vi "Bridge Panel.vi"(8 "error in":errorcluster, 11 "bridge in":T3={"type"=enum."TWM client", "TWM"={"pipe name"="", "parameters"=[], "handle"=0, "fixed aper [s]"=0.0, "f-list [Hz]"=[], "discrete f-list"=FALSE, "unc mode"=enum."None", "unc mcc"=0, "unc first"=FALSE}, "last f"=0.0, "bias comp"={"bias type"=enum."dummy", "VISA"="", "Enable"=FALSE, "channel qu"=[], "channel Uinit"=[]}, "sim mode"=enum."Generic RLC network", "channel idns"=[], "sim phases"=1} {"TWM"."f-list [Hz]" format="%#_6p"}) -> (0 "error out":errorcluster, 3 "bridge out":T3={"type"=enum."TWM client", "TWM"={"pipe name"="", "parameters"=[], "handle"=0, "fixed aper [s]"=0.0, "f-list [Hz]"=[], "discrete f-list"=FALSE, "unc mode"=enum."None", "unc mcc"=0, "unc first"=FALSE}, "last f"=0.0, "bias comp"={"bias type"=enum."dummy", "VISA"="", "Enable"=FALSE, "channel qu"=[], "channel Uinit"=[]}, "sim mode"=enum."Generic RLC network", "channel idns"=[], "sim phases"=1} {"TWM"."f-list [Hz]" format="%#_6p"})   [LabVIEW 2013]
doc: "Bridge configuration panel."
uses:
  Bridge Type.ctl
  Bridge Session.ctl
  drivers/TWM client/TWM Session.ctl
  drivers/TWM client/TWM parameters.ctl
  drivers/TWM client/Meas Proc QWTB Uncertainty Mode.ctl
  Bridge Bias Session.ctl
  Bridge Bias Type.ctl
  Bridge Sim Mode.ctl
  drivers/TWM client.lvlibp/TWM client/TWM Client Algorithm Info.ctl
  drivers/TWM client.lvlibp
  varilib/varilib.lvlib
panel:
  in  "type tc 2":enum32{"dummy"}(tab)
  in  "bias chnc vinit":dbl caption="Channel C: initial voltage [V]" format="%#_6p"
  in  "bias chnb vinit":dbl caption="Channel B: initial voltage [V]" format="%#_6p"
  in  "bias chna vinit":dbl caption="Channel A: initial voltage [V]" format="%#_6p"
  in  "bias chnc qu":string caption="Channel C: quantity name"
  in  "bias chnb qu":string caption="Channel B: quantity name"
  in  "bias chna qu":string caption="Channel A: quantity name"
  in  "bias enable":bool caption="Enable DC bias compensation"
  in  "bias visa":refnum<visa-resource-name> caption="DC bias controller VISA"
  in  "bias type":T1 caption="DC bias controller type"
  out "alginf":T2
  in  "btn cancel":bool
  in  "btn ok":bool
  in  "type tc":enum32{"TWM client", "dummy"}(tab)
  in  "unc first":bool caption="Unc. for 1st reading only"
  in  "unc mcc":i32=1000 caption="Monte carlo cycles" min=1 step=1
  in  "unc mode":T7 caption="Uncertainty calc. mode"
  in  "flist discr":bool caption="Limit fs to discrete list"
  in  "Discrete fs-list [Hz]":dbl[](array[numeric]) format="%#_6p"
  in  "fix aper [s]":dbl caption="Aperture override (0: TWM controlled) [s]" format="%#_3p"
  in  "twm par info":string caption="Parameter description"
  in  "btn twm load":bool
  in  "TWM pipe":string="\\\\.\\pipe\\TWM:server" caption="TWM pipe name (must match TWM server name)"
  in  "twm params":string[][](table) caption="Algorithm parameters"
  in  "sim phase":i32=1 caption="Simulated phase count" min=1 step=1
  in  "sim mode":T9 caption="Simulation mode"
  in  "type":T4 caption="Bridge type"
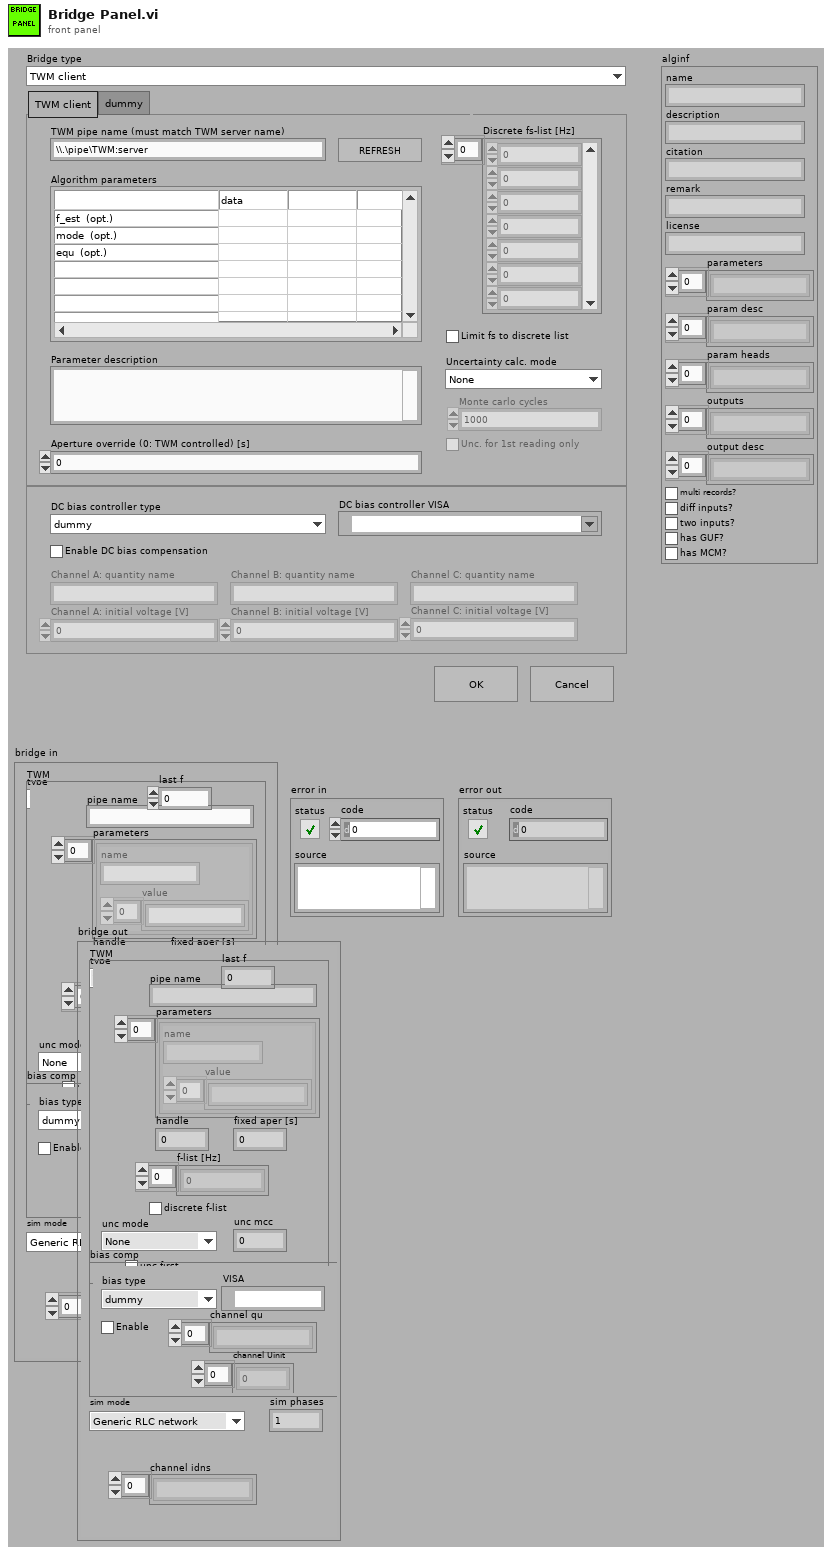
[diagram p1: front panel]
types:
  T1 = typedef "Bridge Bias Type.ctl" = enum16{"dummy", "CMI LiBbias V1.0"}
  T2 = typedef "TWM client.lvlibp/TWM Client Algorithm Info.ctl" = cluster{"name":string, "description":string, "citation":string, "remark":string, "license":string, "parameters":string[], "param desc":string[], "param heads":string[], "outputs":string[], "output desc":string[], "multi records?":bool, "diff inputs?":bool, "two inputs?":bool, "has GUF?":bool, "has MCM?":bool}
  T3 = typedef "Bridge Session.ctl" = cluster{"type":T4, "TWM":T5, "last f":dbl, "bias comp":T8, "sim mode":T9, "channel idns":string[], "sim phases":i32}
  T4 = typedef "Bridge Type.ctl" = enum16{"TWM client", "dummy"}
  T5 = typedef "TWM Session.ctl" = cluster{"pipe name":string, "parameters":T6[], "handle":i32, "fixed aper [s]":dbl, "f-list [Hz]":dbl[], "discrete f-list":bool, "unc mode":T7, "unc mcc":i32, "unc first":bool}
  T6 = typedef "TWM parameters.ctl" = cluster{"name":string, "value":string[]}
  T7 = typedef "Meas Proc QWTB Uncertainty Mode.ctl" = enum16{"None", "GUF", "Monte Carlo"}
  T8 = typedef "Bridge Bias Session.ctl" = cluster{"bias type":T1, "VISA":refnum<visa-resource-name>, "Enable":bool, "channel qu":string[], "channel Uinit":dbl[]}
  T9 = typedef "Bridge Sim Mode.ctl" = enum16{"Generic RLC network", "Interchannel transfer"}
  T10 = typedef "LVRowAndColumnTypeDef.ctl" = cluster{"Row":i32, "Column":i32}
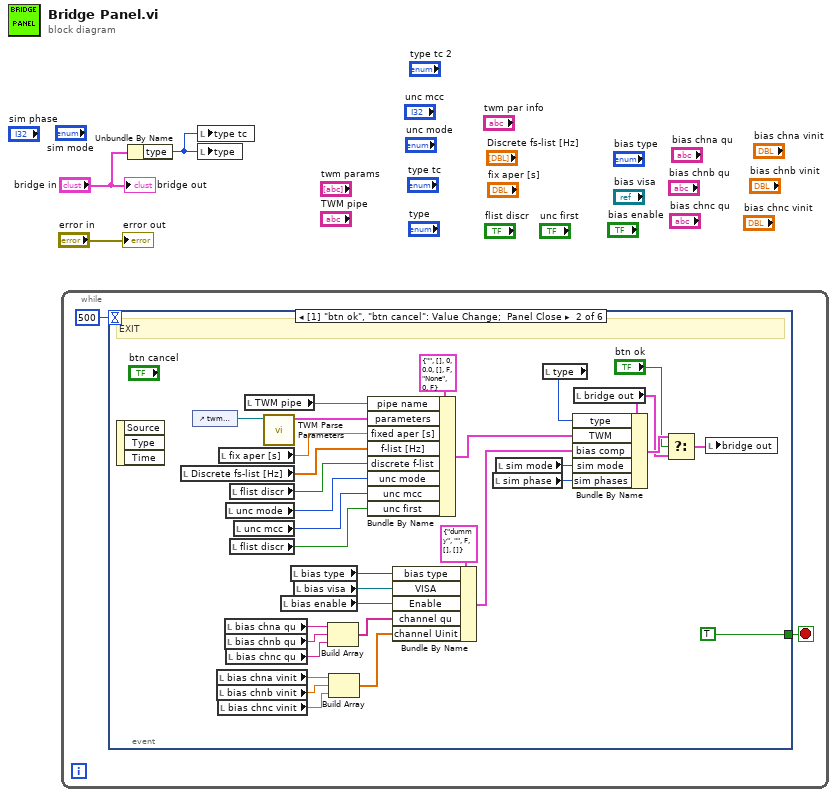
[diagram p0: block diagram]
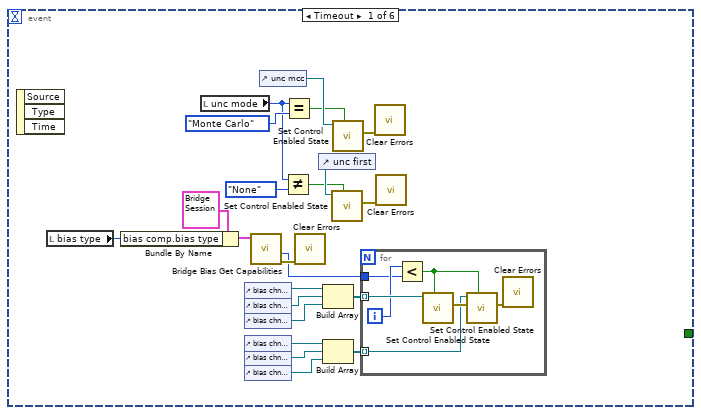
[diagram p2: hidden frame]
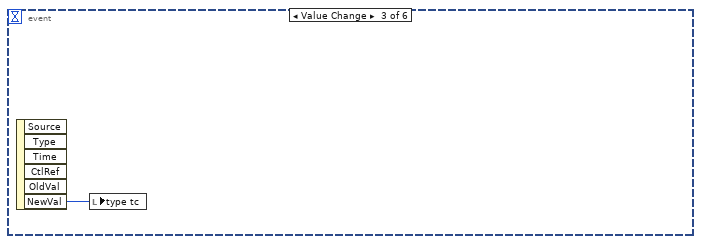
[diagram p3: hidden frame]
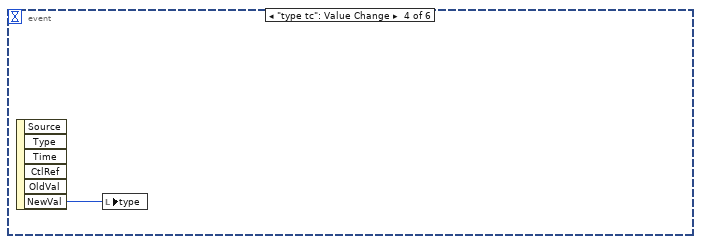
[diagram p4: hidden frame]
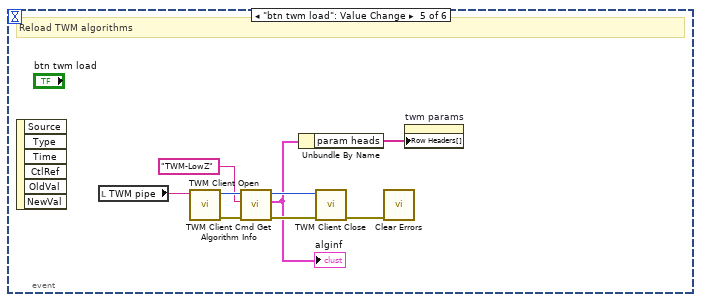
[diagram p5: hidden frame]
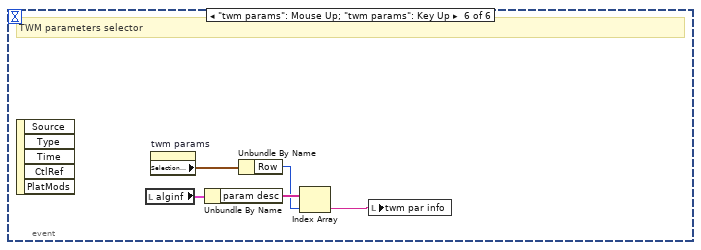
[diagram p6: hidden frame]
diagram:
  n1 = while {
    stop <- w5 stop-if-true
    n2 = event shown="[1] \"btn ok\", \"btn cancel\": Value Change;  Panel Close" {
      selector: _ -> [_ _ _ _ _ _]
      dyn-events: _ -> [_ _ _ _ _ _]
      timeout: 500 -> [_ _ _ _ _ _]
      tunnel: [_ TRUE _ _ _ _] -> w5
      event Timeout {
        n3 = event-data() -> ()  [unwired: 1 in, 3 out]
        n4 = local read "bias type"() -> (w8:T1)
        n5 = Bundle By Name(cluster=T3 {"type"=enum."TWM client", "TWM"={"pipe name"="", "parameters"=[], "handle"=0, "fixed aper [s]"=0.0, "f-list [Hz]"=[], "discrete f-list"=FALSE, "unc mode"=enum."None", "unc mcc"=0, "unc first"=FALSE}, "last f"=0.0, "bias comp"={"bias type"=enum."dummy", "VISA"="", "Enable"=FALSE, "channel qu"=[], "channel Uinit"=[]}, "sim mode"=enum."Generic RLC network", "channel idns"=[], "sim phases"=0} ("bridge session"), "bias comp.bias type"=w8) -> (w10:T3)
        n6 = local read "unc mode"() -> (w19:T7)
        n7 = control-ref of="bias chna qu"() -> (w18:refnum<vi>)
        n8 = control-ref of="bias chnb qu"() -> (w17:refnum<vi>)
        n9 = control-ref of="bias chnc qu"() -> (w16:refnum<vi>)
        n10 = control-ref of="bias chna vinit"() -> (w15:refnum<vi>)
        n11 = control-ref of="bias chnb vinit"() -> (w14:refnum<vi>)
        n12 = control-ref of="bias chnc vinit"() -> (w13:refnum<vi>)
        n13 = call "Bridge Bias Get Capabilities.vi"("bridge in"=w10) -> ("error out"=w7:errorcluster, "channels count"=w6:i32)  [unwired: 7 in, 2 out]
        n14 = control-ref of="unc mcc"() -> (w27:refnum<vi>)
        n15 = Not Equal?(x=w19, y=Meas_Proc_QWTB_Uncertainty_Mode."None") -> (x != y?=w21:bool)
        n16 = Equal?(x=w19, y=Meas_Proc_QWTB_Uncertainty_Mode."Monte Carlo") -> (x = y?=w25:bool)
        n17 = call <vilib>:"Clear Errors.vi"("error in (no error)"=w7) -> ()  [unwired: 6 in, 1 out]
        n18 = control-ref of="unc first"() -> (w23:refnum<vi>)
        n19 = Build Array(w18, w17, w16) -> (w12:refnum<vi>[])
        n20 = Build Array(w15, w14, w13) -> (w11:refnum<vi>[])
        n21 = call "Set Control Enabled State.vi"("enabled (T)"=w21, "reference in"=w23) -> ("error out"=w20:errorcluster)  [unwired: 8 in, 1 out]
        n22 = call "Set Control Enabled State.vi"("enabled (T)"=w25, "reference in"=w27) -> ("error out"=w24:errorcluster)  [unwired: 8 in, 1 out]
        n23 = for {
          tunnel: w12 -> [w34] mode=indexing
          tunnel: w11 -> [w28] mode=indexing
          tunnel: w6 -> [w30]
          i -> [w31]
          n24 = Less?(x=w31, y=w30) -> (x < y?=w29:bool)
          n25 = call "Set Control Enabled State.vi"("enabled (T)"=w29, "reference in"=w34) -> ("error out"=w33:errorcluster)  [unwired: 8 in, 1 out]
          n26 = call "Set Control Enabled State.vi"("enabled (T)"=w29, "error in (no error)"=w33, "reference in"=w28) -> ("error out"=w32:errorcluster)  [unwired: 7 in, 1 out]
          n27 = call <vilib>:"Clear Errors.vi"("error in (no error)"=w32) -> ()  [unwired: 6 in, 1 out]
        }
        n28 = call <vilib>:"Clear Errors.vi"("error in (no error)"=w24) -> ()  [unwired: 6 in, 1 out]
        n29 = call <vilib>:"Clear Errors.vi"("error in (no error)"=w20) -> ()  [unwired: 6 in, 1 out]
      }
      event "btn ok", "btn cancel": Value Change; Panel Close {
        # "EXIT"
        n30 = event-data() -> ()  [unwired: 1 in, 3 out]
        n31 = local read "Discrete fs-list [Hz]"() -> (w55:dbl[])
        n32 = control-ref of="twm params"() -> (w63:refnum<vi>)
        n33 = local read "bias chna vinit"() -> (w40:dbl)
        n34 = local read "bias chnb vinit"() -> (w39:dbl)
        n35 = local read "bias chnc vinit"() -> (w38:dbl)
        n36 = local read "fix aper [s]"() -> (w48:dbl)
        n37 = local read "bias chna qu"() -> (w42:string)
        n38 = local read "bias chnb qu"() -> (w43:string)
        n39 = local read "unc mode"() -> (w53:T7)
        n40 = local read "bias chnc qu"() -> (w44:string)
        n41 = local read "flist discr"() -> (w54:bool)
        n42 = local read "flist discr"() -> (w51:bool)
        n43 = local read "unc mcc"() -> (w52:i32)
        n44 = local read "TWM pipe"() -> (w65:string)
        n45 = call "TWM Parse Parameters.vi"("twm params"=w63) -> ("parameters"=w64:T6[])  [unwired: 9 in, 1 out]
        n46 = local read "bias enable"() -> (w45:bool)
        n47 = local read "bias type"() -> (w47:T1)
        n48 = local read "bias visa"() -> (w46:refnum<visa-resource-name>)
        n49 = Build Array(w42, w43, w44) -> (w41:string[])
        n50 = Build Array(w40, w39, w38) -> (w37:dbl[])
        n51 = Bundle By Name(cluster=T5 {"pipe name"="", "parameters"=[], "handle"=0, "fixed aper [s]"=0.0, "f-list [Hz]"=[], "discrete f-list"=FALSE, "unc mode"=enum."None", "unc mcc"=0, "unc first"=FALSE} ("TWM cfg"), "pipe name"=w65, "parameters"=w64, "fixed aper [s]"=w48, "f-list [Hz]"=w55, "discrete f-list"=w54, "unc mode"=w53, "unc mcc"=w52, "unc first"=w51) -> (w61:T5)
        n52 = Bundle By Name(cluster=T8 {"bias type"=enum."dummy", "VISA"="", "Enable"=FALSE, "channel qu"=[], "channel Uinit"=[]} ("bias comp"), "bias type"=w47, "VISA"=w46, "Enable"=w45, "channel qu"=w41, "channel Uinit"=w37) -> (w49:T8)
        n53 = local read "sim phase"() -> (w35:i32)
        n54 = local read "sim mode"() -> (w36:T9)
        n55 = local read "type"() -> (w62:T4)
        n56 = local read "bridge out"() -> (w59:T3)
        n57 = Bundle By Name(cluster=w59, "type"=w62, "TWM"=w61, "bias comp"=w49, "sim mode"=w36, "sim phases"=w35) -> (w60:T3)
        n58 = Select(t=w60, s="btn ok", f=w59) -> (s? t:f=w58:T3)
        n59 = local write "bridge out"(w58) -> ()
      }
      event Value Change {
        n60 = event-data() -> ("NewVal"=w67:T4)  [unwired: 1 in, 5 out]
        n61 = local write "type tc"(w67) -> ()
      }
      event "type tc": Value Change {
        n62 = event-data() -> ("NewVal"=w68:enum32{"TWM client", "dummy"})  [unwired: 1 in, 5 out]
        n63 = local write "type"(w68) -> ()
      }
      event "btn twm load": Value Change {
        # "Reload TWM algorithms"
        n64 = event-data() -> ()  [unwired: 1 in, 6 out]
        n65 = local read "TWM pipe"() -> (w73:string)
        n66 = call "TWM Client Open.vi"("pipe name"=w73) -> ("error out"=w77:errorcluster, "handle out"=w76:i32)  [unwired: 9 in]
        n67 = call "TWM Client Cmd Get Algorithm Info.vi"("error in"=w77, "algorithm id"="TWM-LowZ" ("multi-line string"), "handle"=w76) -> ("error out"=w74:errorcluster, "algorithm info"=w71:T2, "handle out"=w75:i32)  [unwired: 6 in]
        "alginf" <- w71
        n68 = Unbundle By Name(w71) -> ("param heads"=w70:string[])
        n69 = call "TWM Client Close.vi"("error in"=w74, "handle in"=w75) -> ("error out"=w72:errorcluster)  [unwired: 9 in]
        n70 = call <vilib>:"Clear Errors.vi"("error in (no error)"=w72) -> ()  [unwired: 6 in, 1 out]
        n71 = property on="twm params" class="Tbl (strict)"("Row Headers[]"=w70) -> ()  [unwired: 2 in, 2 out]
      }
      event "twm params": Mouse Up; "twm params": Key Up {
        # "TWM parameters selector"
        n72 = event-data() -> ()  [unwired: 1 in, 5 out]
        n73 = local read "alginf"() -> (w82:T2)
        n74 = property on="twm params" class="Tbl (strict)"() -> ("Selection Start"=w81:T10)  [unwired: 2 in, 2 out]
        n75 = Unbundle By Name(w82) -> ("param desc"=w80:string[])
        n76 = Unbundle By Name(w81) -> ("Row"=w79:i32)
        n77 = Index Array(array=w80, index=w79) -> (element=w78:string)
        n78 = local write "twm par info"(w78) -> ()
      }
    }
  }
  n79 = Unbundle By Name("bridge in") -> ("type"=w1:T4)
  n80 = local write "type tc"(w1) -> ()
  n81 = local write "type"(w1) -> ()
  "error out" <- "error in"
  "bridge out" <- "bridge in"
